vi "Scanning Status.vi"(10 "Ready to Scan":bool, 11 "Done out":bool) -> (3 "Status out":enum16{"Waiting", "Scanning", "Stop"}(ring))   [LabVIEW 2015]
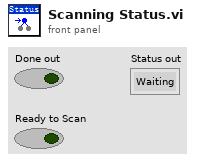
[diagram p1: front panel]
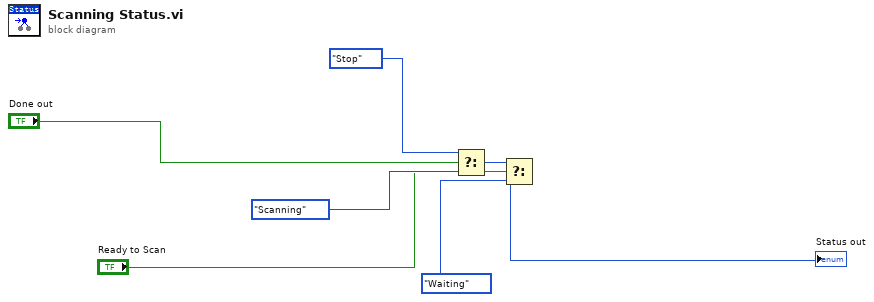
[diagram p0: block diagram]
diagram:
  n1 = Select(t=enum16{"Waiting", "Scanning", "Stop"}."Stop", s="Done out", f=enum16{"Waiting", "Scanning", "Stop"}."Scanning") -> (s? t:f=w6:enum16{"Waiting", "Scanning", "Stop"})
  n2 = Select(t=w6, s="Ready to Scan", f=enum16{"Waiting", "Scanning", "Stop"}."Waiting") -> (s? t:f=→"Status out":enum16{"Waiting", "Scanning", "Stop"})
